vi "Feeder_Motor_global.vi"() -> ()   [LabVIEW 2020]
uses:
  Feeder_Cluster.ctl
  Subsystems/Funnel/Funnel_Cluster.ctl
  Subsystems/Funnel/Control_States_Funnel.ctl
  Subsystems/Intake/Intake_cluster.ctl
  Subsystems/Intake/Intake_control_states.ctl
  Subsystems/Magazine/Magazine_Cluster.ctl
  Subsystems/Magazine/Magazine_Control_States.ctl
panel:
  in  "Feeder_Set_Notifier":refnum<notifier>
  in  "Feeder_Set_Ref":string="Feeder_Set_Ref"
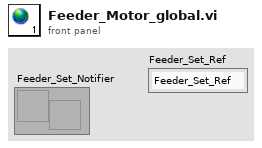
[diagram p1: front panel]
diagram:
